vi "Obtain.vi"(10 "Alias":string) -> (0 "error out":errorcluster, 2 "Msg Q":refnum<data-value>)   [LabVIEW 2021, in "LVCAM.lvlib" / "Msg Q.lvclass"]
uses:
  Msg Q.lvclass
  Msg/Msg.lvclass
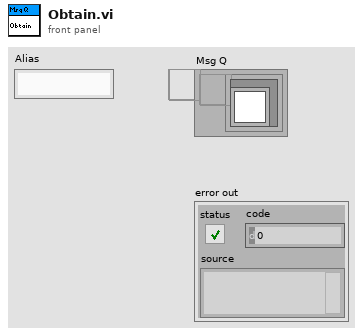
[diagram p1: front panel]
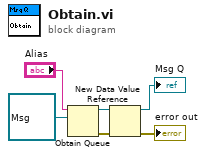
[diagram p0: block diagram]
diagram:
  n1 = Obtain Queue(name (unnamed)="Alias", element data type=refnum<class "Msg.lvclass"> refnum ("Artifex Actor Model.lvlib:Msg.lvclass")) -> (queue out=w3:refnum<queue>, error out=w6:errorcluster)  [unwired: 3 in, 1 out]
  n2 = New Data Value Reference(data value=w3, error in=w6) -> (data value reference=→"Msg Q":refnum<data-value>, error out=→"error out":errorcluster)
